vi "day 12 task 1.vi"() -> ()   [LabVIEW 2019]
panel:
  out "Array 2":bool[](array[boolean])
  out "Array":bool[](array[boolean])
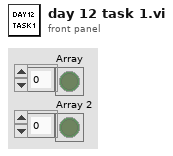
[diagram p1: front panel]
types:
  T1 = cluster{"current location":cluster{"x":i32, "y":i32}, "goal location":cluster{"x":i32, "y":i32}, "visited":bool[][], "heightmap":u8[][], "lettermap":string[][], "visited":cluster{"x":i32, "y":i32}[]}
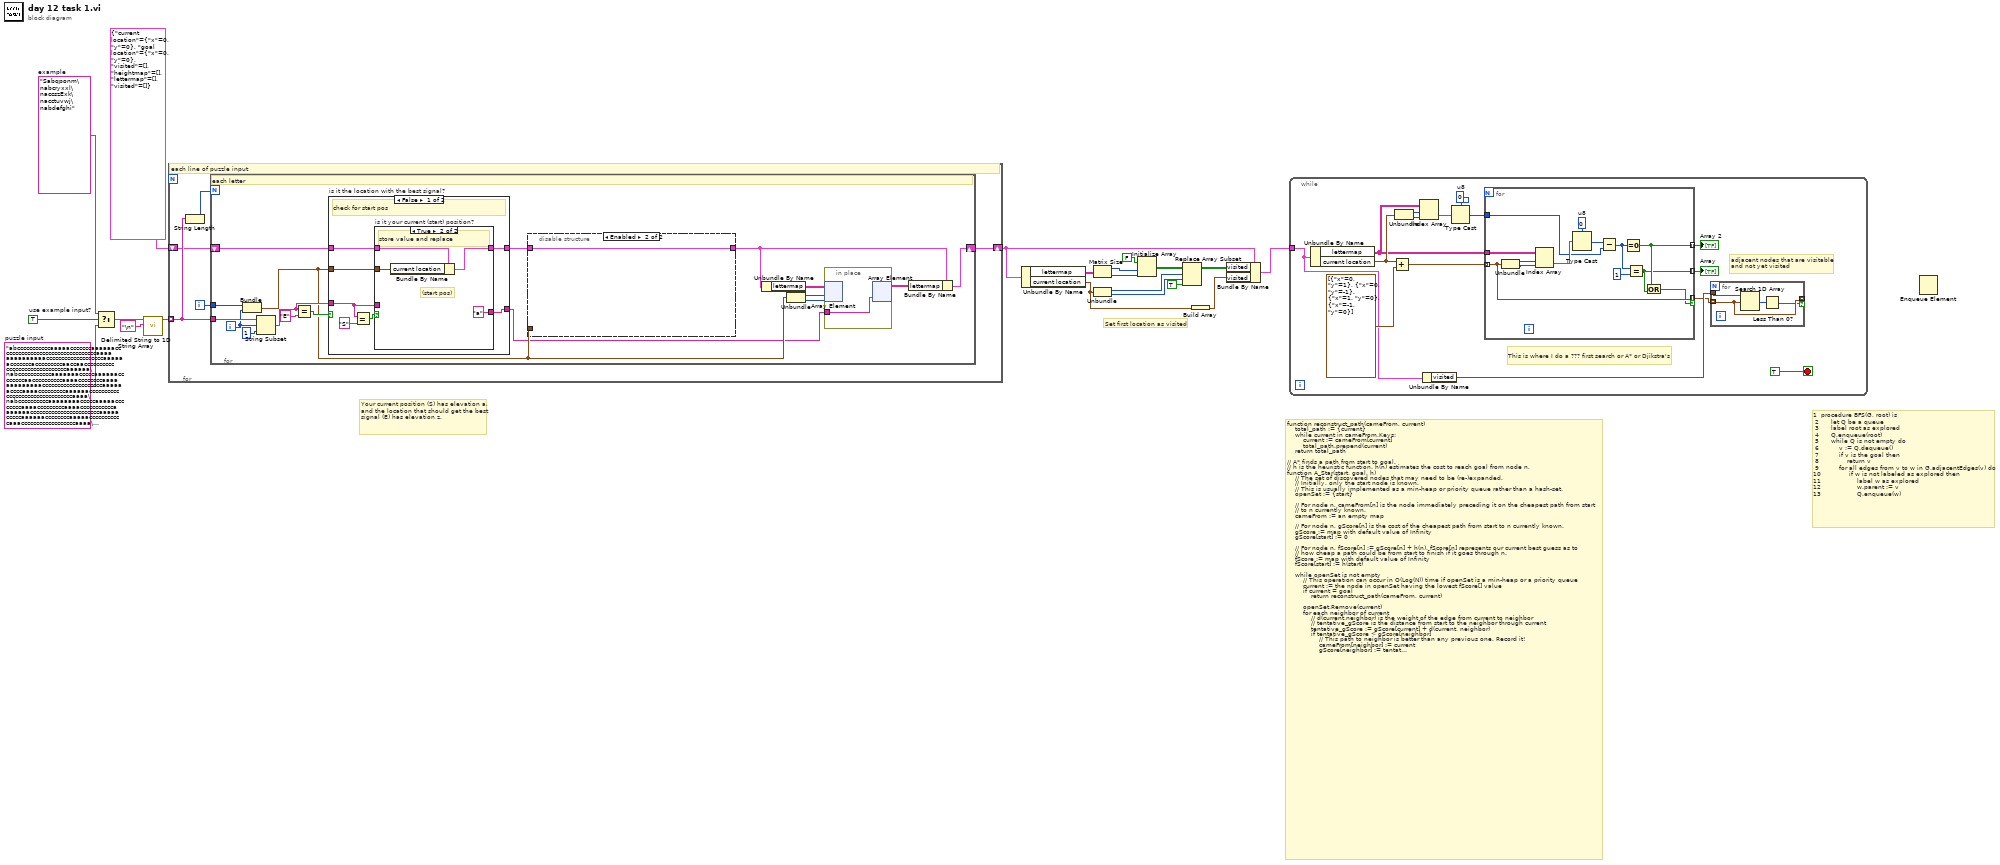
[diagram p0: block diagram]
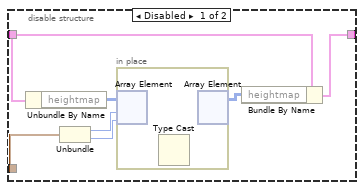
[diagram p2: hidden frame]
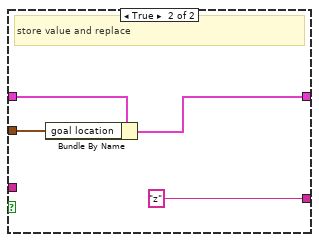
[diagram p4: hidden frame]
diagram:
  w18 = "Sabqponm\nabcryxxl\naccszExk\nacctuvwj\nabdefghi"  # example
  w19 = TRUE  # use example input?
  w20 = "abcccccccccccaaaaacccccccaaaaaaccccccccccccccccccccccccccccccccaaaaaaaaaaaaaacccccccccccccccccccaaaaaacccccccacccccccccaaccaaccccccccccccccccccccccccccccccaaaaaa\nabcccccccccccaaaaaaacccccaaaaaaccccccccaaccccccccccaaaaccccccccaaaaaaaaaaaaaccccccccccccccccccccaaaaaaccccaaaacccccccccaaaaaaccccccccccccccccccccccccccccccccaaaa\nabccccccccccaaaaaaaacccccaaaaaccccccccaaaacccccccccaaaacccccccccccaaaaaaacccccccccccccccccccccccaaaaacccccaaaaaaccccccccaaaaacccccccccccaaaccccccccccccccccccaaaa\nabccccccccccaaaaaaaaccccccaaaaacccccccaaaacccccccccaaaacccccaaaccccaaaaaaccccccccccccccccccccccccaaaaacccccaaaaacc..."  # puzzle input
  # "1  procedure BFS(G, root) is\n 2      let Q be a queue\n 3      label root as explored\n 4      Q.enqueue(root)\n 5      while Q is not empty do\n 6          v := Q.dequeue()\n 7          if v is the goal then\n 8              return v\n 9          for all edges from v to w in G.adjacentEdges(v) do\n10              if w is not labeled as explored then\n11                  label w as explored\n12                  w.parent := v\n13                  Q.enqueue(w)"
  # "function reconstruct_path(cameFrom, current)\n    total_path := {current}\n    while current in cameFrom.Keys:\n        current := cameFrom[current]\n        total_path.prepend(current)\n    return total_path\n\n// A* finds a path from start to goal.\n// h is the heuristic function. h(n) estimates the cost to reach goal from node n.\nfunction A_Star(start, goal, h)\n    // The set of discovered nodes that may need to be (re-)expanded.\n    // Initially, only the start node is known.\n    // This is usually implemented as a min-heap or priority queue rather than a hash-set.\n    openSet := {start}\n\n    // For node n, cameFrom[n] is the node immediately preceding it on the cheapest path from start\n    // to n currently known.\n    cameFrom := an empty map\n\n    // For node n, gScore[n] is the cost of the cheapest path from start to n currently known.\n    gScore := map with default value of Infinity\n    gScore[start] := 0\n\n    // For node n, fScore[n] := gScore[n] + h(n). fScore[n] represents our current best guess as to\n    // how cheap a path could be from start to finish if it goes through n.\n    fScore := map with default value of Infinity\n    fScore[start] := h(start)\n\n    while openSet is not empty\n        // This operation can occur in O(Log(N)) time if openSet is a min-heap or a priority queue\n        current := the node in openSet having the lowest fScore[] value\n        if current = goal\n            return reconstruct_path(cameFrom, current)\n\n        openSet.Remove(current)\n        for each neighbor of current\n            // d(current,neighbor) is the weight of the edge from current to neighbor\n            // tentative_gScore is the distance from start to the neighbor through current\n            tentative_gScore := gScore[current] + d(current, neighbor)\n            if tentative_gScore < gScore[neighbor]\n                // This path to neighbor is better than any previous one. Record it!\n                cameFrom[neighbor] := current\n                gScore[neighbor] := tentative_gScore\n                fScore[neighbor] := tentative_gScore + h(neighbor)\n                if neighbor not in openSet\n                    openSet.add(neighbor)\n\n    // Open set is empty but goal was never reached\n    return failure"
  # "Set first location as visited"
  # "Your current position (S) has elevation a, and the location that should get the best signal (E) has elevation z."
  n1 = Select(t=w18, s=w19, f=w20) -> (s? t:f=w17:string)
  n2 = call <vilib>:"Delimited String to 1D String Array.vi"("delimiter"="\n" ("regular expression"), "delimited string"=w17) -> ("string array"=w15:string[])  [unwired: 9 in]
  n3 = for {
    tunnel: w15 -> [w24] mode=indexing
    shift-right: [w22] -> w5
    shift-left: T1 {"current location"={"x"=0, "y"=0}, "goal location"={"x"=0, "y"=0}, "visited"=[], "heightmap"=[], "lettermap"=[], "visited"=[]} -> [w21]
    i -> [w23]
    # "each line of puzzle input"
    n4 = String Length(string=w24) -> (length=w25:i32)
    n5 = for {
      N: w25 -> [_]
      tunnel: w24 -> [w41]
      tunnel: w23 -> [w38]
      shift-right: [w26] -> w22
      shift-left: w21 -> [w36]
      i -> [w39]
      # "each letter"
      n6 = Bundle(w38, w39) -> (w34:cluster{i32, i32})  [unwired: 1 in]
      n7 = String Subset(string=w41, offset (0)=w39, length (rest)=1 ("length (rest)")) -> (substring=w35:string)
      n8 = Equal?(x=w35, y="E") -> (x = y?=w37:bool)
      n9 = case "is it the location with the best signal?" shown="False" w37 {
        tunnel: w36 -> [w56 w68]
        tunnel: w34 -> [w55 w67]
        tunnel: [w54 w66] -> w31
        tunnel: w35 -> [w52 _]
        tunnel: [w53 "z" ("y")] -> w29
        frame False {
          # "check for start pos"
          n10 = Equal?(x=w52, y="S") -> (x = y?=w57:bool)
          n11 = case "is it your current (start) position?" shown="True" w57 {
            tunnel: w56 -> [w60 w64]
            tunnel: w55 -> [_ w63]
            tunnel: [w60 w62] -> w54
            tunnel: [w59 "a" ("String")] -> w53
            tunnel: w52 -> [w59 _]
            frame False {
              # "just pass the letter through"
            }
            frame True {
              # "(start pos)"
              # "store value and replace"
              n12 = Bundle By Name(cluster=w64, "current location"=w63) -> (w62:T1)
            }
          }
        }
        frame True {
          # "store value and replace"
          n13 = Bundle By Name(cluster=w68, "goal location"=w67) -> (w66:T1)
        }
      }
      n14 = disable-structure shown="Enabled" {
        disable-tunnel: w34 -> [w46 _]
        disable-tunnel: w31 -> [w45 w50]
        disable-tunnel: [w44 w50] -> w27
        frame Disabled {
          n15 = Unbundle By Name(w45) -> ("heightmap"=w49:u8[][])
          n16 = Unbundle(w46) -> (w48:i32, w47:i32)
          n17 = in-place {
            n18 = in-place-array #1(w49, w48, w47) -> ()  [unwired: 1 out]
            n19 = Type Cast() -> ()  [unwired: 2 in, 1 out]
            n20 = in-place-array #1() -> (w43:u8[][])  [unwired: 1 in, 2 out]
          }
          n21 = Bundle By Name(cluster=w45, "heightmap"=w43) -> (w44:T1)
        }
        frame Enabled {
        }
      }
      n22 = Unbundle By Name(w27) -> ("lettermap"=w30:string[][])
      n23 = Unbundle(w34) -> (w33:i32, w32:i32)
      n24 = in-place {
        in-place-border: w29 -> [w51]
        n25 = in-place-array #2(w30, w33, w32) -> ()  [unwired: 1 out]
        n26 = in-place-array #2(w51) -> (w28:string[][])  [unwired: 2 out]
      }
      n27 = Bundle By Name(cluster=w27, "lettermap"=w28) -> (w26:T1)
    }
  }
  n28 = Unbundle By Name(w5) -> ("lettermap"=w13:string[][], "current location"=w1:cluster{"x":i32, "y":i32})
  n29 = Matrix Size(0:w13) -> (1:w11:i32, 2:w10:i32)
  n30 = Unbundle(w1) -> ("x"=w8:i32, "y"=w7:i32)
  n31 = Initialize Array(FALSE, w11, w10) -> (w9:bool[][])
  n32 = Replace Array Subset(array=w9, new element=TRUE, index (row)=w8, index (col)=w7) -> (w3:bool[][])
  n33 = Build Array(w1) -> (w2:cluster{"x":i32, "y":i32}[])
  n34 = Bundle By Name(cluster=w5, "visited"=w3, "visited"=w2) -> (w4:T1)
  n35 = while {
    tunnel: w4 -> [w71]
    stop <- TRUE stop-if-true
    w75 = u8 0  # u8
    # "adjacent nodes that are visitable\nand not yet visited"
    # "This is where I do a ??? first search or A* or Djikstra's"
    n36 = Unbundle By Name(w71) -> ("lettermap"=w77:string[][], "current location"=w80:cluster{"x":i32, "y":i32})
    n37 = Add(x=w80, y=cluster{"x":i32, "y":i32}[] [{"x"=0, "y"=1}, {"x"=0, "y"=-1}, {"x"=1, "y"=0}, {"x"=-1, "y"=0}]) -> (x+y=w81:cluster{"x":i32, "y":i32}[])
    n38 = Unbundle(w80) -> ("x"=w79:i32, "y"=w78:i32)
    n39 = Index Array(array=w77, index (row)=w79, index (col)=w78) -> (element=w76:string)
    n40 = Unbundle By Name(w71) -> ("visited"=w70:cluster{"x":i32, "y":i32}[])
    n41 = Type Cast(type=w75, x=w76) -> (*(type *) &x=w74:u8)
    n42 = for {
      tunnel: w77 -> [w100]
      tunnel: w81 -> [w91] mode=indexing
      tunnel: w74 -> [w94]
      tunnel: [w90] -> w72 mode=indexing
      tunnel: [w89] -> w73 mode=indexing
      tunnel: [w91] -> w69 mode=indexing if=w88
      w97 = u8 0  # u8
      n43 = Unbundle(w91) -> ("x"=w99:i32, "y"=w98:i32)
      n44 = Index Array(array=w100, index (row)=w99, index (col)=w98) -> (element=w96:string)
      n45 = Type Cast(type=w97, x=w96) -> (*(type *) &x=w95:u8)
      n46 = Subtract(x=w95, y=w94) -> (x-y=w93:u8)
      n47 = Equal To 0?(x=w93) -> (x = 0?=w90:bool)
      n48 = Equal?(x=w93, y=u8 1) -> (x = y?=w89:bool)
      n49 = Or(x=w90, y=w89) -> (x .or. y?=w88:bool)
    }
    "Array" <- w73
    "Array 2" <- w72
    n50 = for {
      tunnel: w70 -> [w87]
      tunnel: w69 -> [w85] mode=indexing
      tunnel: [w85] -> _ mode=indexing if=w84
      n51 = Search 1D Array(1D array=w87, element=w85) -> (index of element=w86:i32)  [unwired: 1 in]
      n52 = Less Than 0?(x=w86) -> (x < 0?=w84:bool)
    }
  }
  n53 = Enqueue Element() -> ()  [unwired: 4 in, 3 out]
